vi "Send Receive Usb Command.vi"(8 "error in (no error)":errorcluster, 10 "MaxResponseTime":u32=100, 11 "Cmd in":u8[](array[numeric])) -> (0 "error out":errorcluster, 1 "Return":u32, 2 "RecvLength out":u32, 3 "Cmd out":u8[](array[numeric]))   [LabVIEW 2010, in "TPVG_DLL.lvlib"]
doc: "This function must be called to send a command to the usb device and wait for a valide and verified anwser\n\n\n\nDWORD CLASS_DECLSPEC SendReceiveUsbCommand( BYTE*, DWORD*, DWORD );"
uses:
  TPVG_DLL.lvlib
  TPVG_DLL.dll
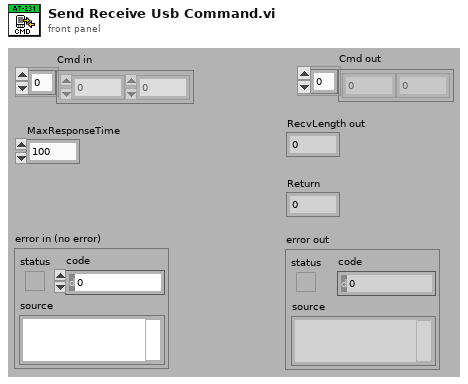
[diagram p1: front panel]
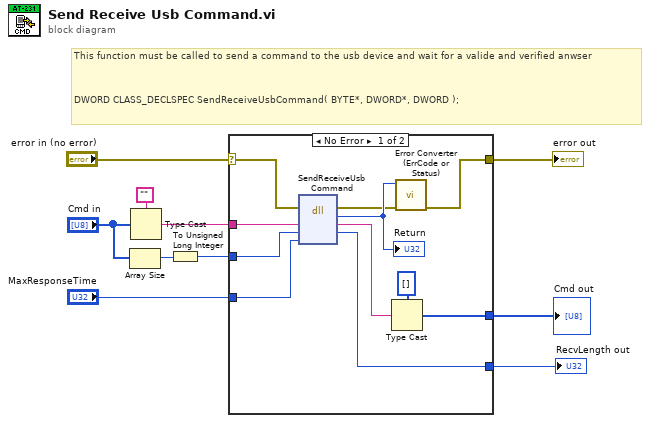
[diagram p0: block diagram]
diagram:
  # "This function must be called to send a command to the usb device and wait for a valide and verified anwser\n\n\n\nDWORD CLASS_DECLSPEC SendReceiveUsbCommand( BYTE*, DWORD*, DWORD );"
  n1 = Array Size(array="Cmd in") -> (size(s)=w5:i32)
  n2 = Type Cast(type="", x="Cmd in") -> (*(type *) &x=w7:string)
  n3 = To Unsigned Long Integer(number=w5) -> (unsigned 32bit integer=w4:u32)
  n4 = case shown="No Error" "error in (no error)" {
    selector: "error in (no error)" -> [w12 w22]
    tunnel: [w20 _] -> w10
    tunnel: "MaxResponseTime" -> [w19 _]
    tunnel: w7 -> [w17 _]
    tunnel: w4 -> [w16 _]
    tunnel: [w13 _] -> w3
    tunnel: [w11 w22] -> w1
    frame No Error {
      n5 = dll-call lib="TPVG_DLL.dll" fn="SendReceiveUsbCommand"(error in=w12, "RecvBuffer"=w17, "RecvLength"=w16, "MaxResponseTime"=w19) -> (error out=w18:errorcluster, "return type"=w21:u32, "RecvBuffer"=w15:string, "RecvLength"=w20:u32)  [unwired: 3 in, 1 out]
      "Return" <- w21
      n6 = Type Cast(type=u8[] [], x=w15) -> (*(type *) &x=w13:u8[])
      n7 = call "Error Converter (ErrCode or Status).vi"("error in (no error)"=w18, "error code"=w21) -> ("error out"=w11:errorcluster)  [unwired: 9 in]
    }
    frame Error {
    }
  }
  "RecvLength out" <- w10
  "error out" <- w1
  "Cmd out" <- w3
